vi "Set Symbol.vi"(7 "error in (no error)":errorcluster, 8 "ItemName":string, 10 "Popup Listbox In":refnum<vi>) -> (0 "error out":errorcluster, 3 "Popup Listbox Out":refnum<vi>)   [LabVIEW 2012]
uses:
  ListBox/Custom Type/Read and Write Mode.ctl
  ListBox/Property/Set and Get ItemNames.vi
  ListBox/Property/Set and Get ItemNames With Symbol.vi
  ListBox/Listbox Tool.lvlib
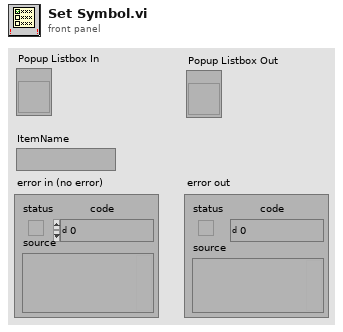
[diagram p1: front panel]
types:
  T1 = typedef "Listbox Tool.lvlib/Read and Write Mode.ctl" = enum16{"Read", "Write"}
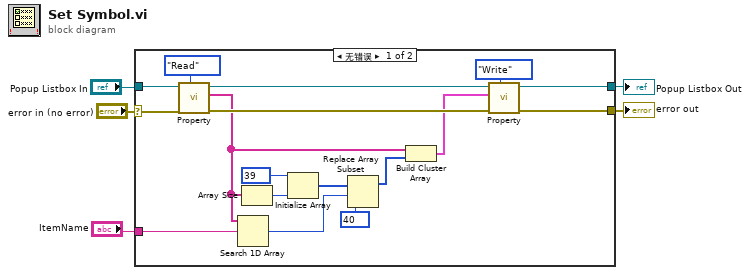
[diagram p0: block diagram]
diagram:
  n1 = case shown="无错误" "error in (no error)" {
    selector: "error in (no error)" -> [w21 w24]
    tunnel: [w7 w24] -> w4
    tunnel: "Popup Listbox In" -> [w22 w23]
    tunnel: "ItemName" -> [w15 _]
    tunnel: [w8 w23] -> w1
    frame No Error {
      n2 = call-poly "Property.vi"("Mode"=Read_and_Write_Mode."Read", "错误输入"=w21, "Listbox Ref"=w22) -> ("错误输出"=w19:errorcluster, "ItemNames Out"=w11:string[], "Dup Listbox Ref"=w18:refnum<vi>)  [unwired: 6 in]
      n3 = Search 1D Array(1D array=w11, element=w15) -> (index of element=w13:i32)  [unwired: 1 in]
      n4 = Array Size(array=w11) -> (size(s)=w16:i32)
      n5 = Initialize Array(39, w16) -> (w14:i32[])
      n6 = Replace Array Subset(array=w14, new element=40, index=w13) -> (w10:i32[])
      n7 = Build Cluster Array(w11, w10) -> (w6:cluster{"字符串":string, i32}[])
      n8 = call-poly "Property.vi"("Mode"=Read_and_Write_Mode."Write", "错误输入"=w19, "ItemNames In"=w6, "Listbox Ref"=w18) -> ("错误输出"=w7:errorcluster, "Dup Listbox Ref"=w8:refnum<vi>)  [unwired: 5 in, 1 out]
    }
    frame Error {
    }
  }
  "error out" <- w4
  "Popup Listbox Out" <- w1
